vi "Record.vi"() -> ()   [LabVIEW 2010]
uses:
  <vilib>/userDefined/High Color/IMAQdx.ctl
  <vilib>/vision/driver/NI_Vision_Acquisition_Software.lvlib
panel:
  out "Data":dynamicdata(graph)
  out "Image":T1(plugin-control)
  in  "Duration":u32=30
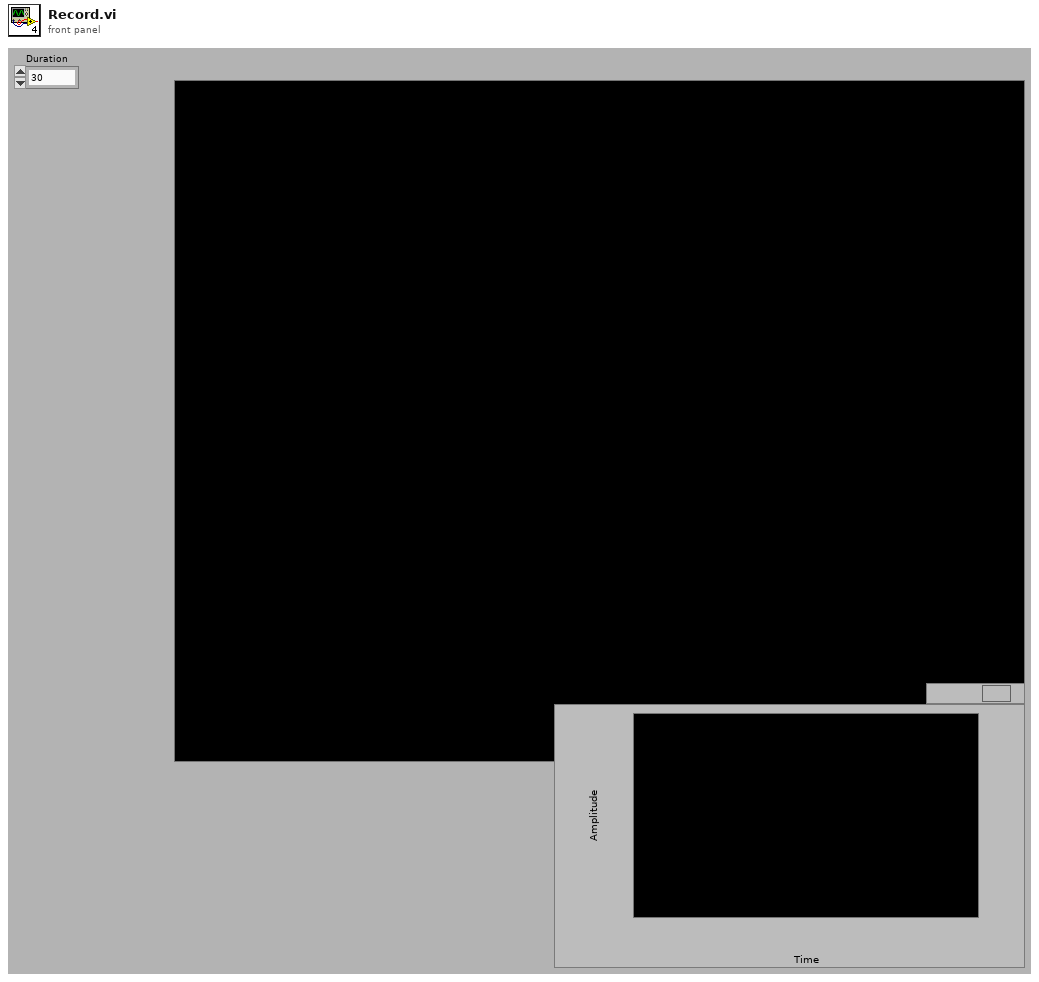
[diagram p1: front panel]
types:
  T1 = typedef "IMAQ Image.ctl" = refnum<image>
  T2 = typedef "Image Type" = u32
  T3 = typedef "IMAQdx.ctl" = refnum<k21>
  T4 = typedef "AviRefnum.ctl" = refnum<k1>
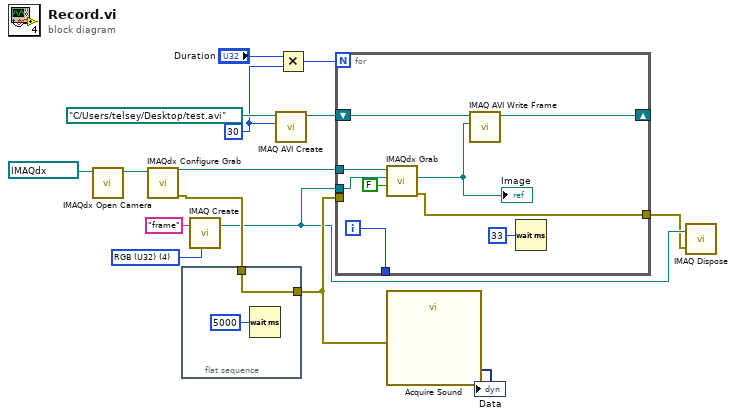
[diagram p0: block diagram]
diagram:
  w3 = T2 4 items=["Grayscale (U8)", "Grayscale (I16)", "Grayscale (SGL)", "Complex (CSG)", "RGB (U32)", "HSL (U32)", "RGB (U64)", "Grayscale (U16)"] ("Image Type")
  w13 = u32 30 ("Frames Per Second")
  n1 = call <vilib>:"IMAQdx Open Camera.vi"("Session In"=T3 "webcam") -> ("Session Out"=w10:T3)  [unwired: 9 in, 1 out]
  n2 = call <vilib>:"IMAQdx Configure Grab.vi"("Session In"=w10) -> ("error out"=w6:errorcluster, "Session Out"=w9:T3)  [unwired: 9 in]
  n3 = flat-sequence {
    tunnel: [w16] -> w5
    tunnel: w6 -> [w16]
    frame #0 {
      n4 = Wait (ms)(milliseconds to wait=u32 5000) -> ()  [unwired: 1 out]
    }
  }
  n5 = call "IMAQ Create"("Image Name"="frame", "Image Type"=w3) -> ("New Image"=w2:T1)  [unwired: 3 in, 1 out]
  n6 = call "IMAQ AVI Create"("Frames Per Second"=w13, "AVI Path"=path "C:/Users/telsey/Desktop/test.avi") -> ("Avi Refnum"=w7:T4)  [unwired: 8 in, 1 out]
  n7 = Multiply(x="Duration", y=w13) -> (x*y=w14:u32)
  n8 = for {
    N: w14 -> [_]
    tunnel: w9 -> [w26]
    tunnel: w2 -> [w25]
    shift-right: [w22] -> _
    shift-left: w7 -> [w23]
    tunnel: w5 -> [_]
    tunnel: [w20] -> _
    tunnel: [w18] -> w1
    i -> [w20]
    n9 = call <vilib>:"IMAQdx Grab.vi"("Wait for Next Buffer? (Yes)"=FALSE, "Image In"=w25, "Session In"=w26) -> ("error out"=w18:errorcluster, "Image Out"=w21:T1)  [unwired: 5 in, 2 out]
    "Image" <- w21
    n10 = call "IMAQ AVI Write Frame"("Image"=w21, "Avi Refnum"=w23) -> ("Avi Refnum (duplicate)"=w22:T4)  [unwired: 8 in, 1 out]
    n11 = Wait (ms)(milliseconds to wait=u32 33) -> ()  [unwired: 1 out]
  }
  n12 = call "Acquire Sound"("error in (no error)"=w5) -> ("Data"=→"Data":dynamicdata)  [unwired: 17 in, 1 out]
  n13 = call "IMAQ Dispose"("Image"=w2, "error in (no error)"=w1) -> ()  [unwired: 4 in, 1 out]
